vi "QI_ListCam.vi"(8 "error in (no error)":errorcluster, 11 "path to dll":path) -> (0 "error out":errorcluster, 1 "LibCam Error":u32, 2 "cameraId":u32)   [LabVIEW 2014]
panel:
  out "listLength":u32
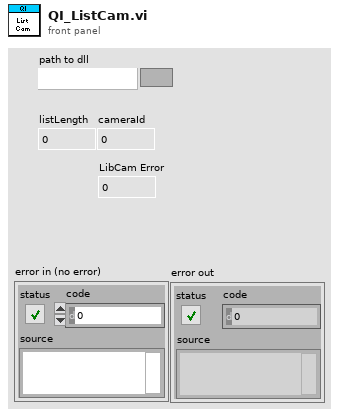
[diagram p1: front panel]
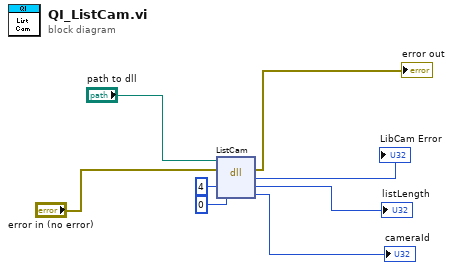
[diagram p0: block diagram]
diagram:
  n1 = dll-call lib="C:/Users/appli/Documents/Aline/octo-labview/QImaging/Release/QImaging.dll" fn="ListCam"(path in="path to dll", error in="error in (no error)", "listLength"=u32 4, "cameraId"=u32 0) -> (error out=→"error out":errorcluster, "return type"=→"LibCam Error":u32, "listLength"=→"listLength":u32, "cameraId"=→"cameraId":u32)  [unwired: 1 in, 1 out]
